vi "Arcade Drive.vi"(8 "b":dbl=1.0, 9 "a":dbl=1.0, 10 "turn":dbl, 11 "throttle":dbl) -> (2 "right power":dbl, 3 "left power":dbl)   [LabVIEW 2014]
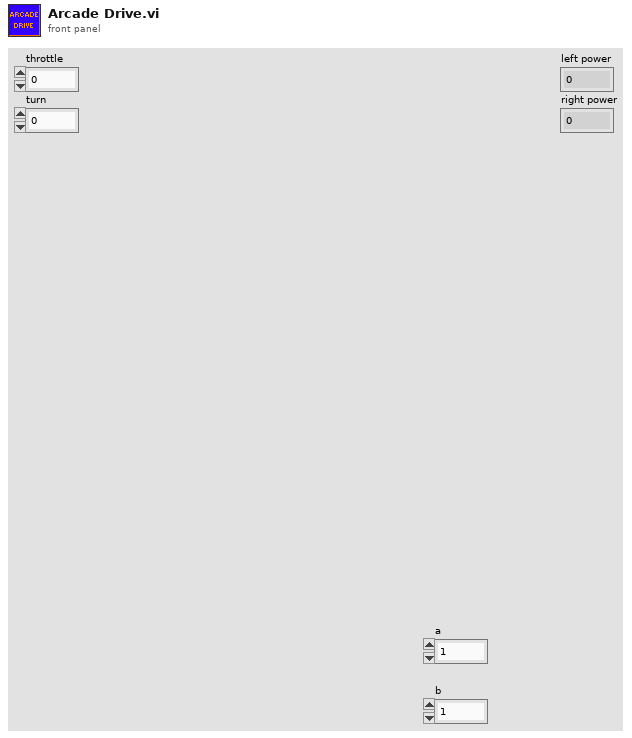
[diagram p1: front panel]
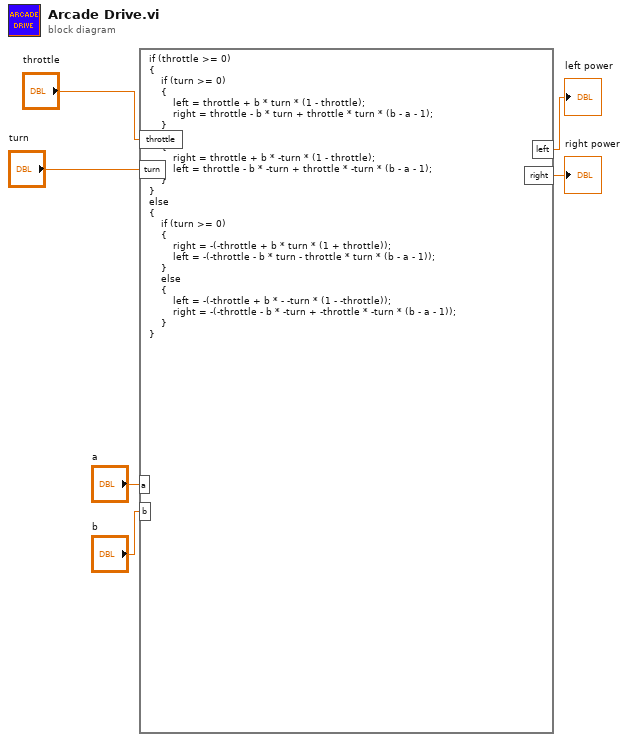
[diagram p0: block diagram]
diagram:
  n1 = formula code="if (throttle >= 0)\n{\n    if (turn >= 0)\n    {\n        left = throttle + b * turn * (1 - throttle);\n        right = throttle - b * turn + throttle * turn * (b - a - 1);\n    }\n    else\n    {\n        right = throttle + b * -turn * (1 - throttle);\n        left = throttle - b * -turn + throttle * -turn * (b - a - 1);\n    }\n}\nelse\n{\n    if (turn >= 0)\n    {\n        right = -(-throttle + b * turn * (1 + throttle));\n        left = -(-throttle - b * turn - throttle * turn * (b - a - 1));\n    }\n    else\n    {\n        left = -(-throttle + b * - -turn * (1 - -throttle));\n        right = -(-throttle - b * -turn + -throttle * -turn * (b - a - 1));\n    }\n}"("throttle"="throttle", "turn"="turn", "a"="a", "b"="b") -> ("left"=→"left power":dbl, "right"=→"right power":dbl)
